vi "XIPIN_AXI_BFM_Cores_5_0.vi"   [LabVIEW 2017]
doc: "Cadence Axi BFM Cores\n------------------------------------\n<b>Need License</b> : Yes\n<b>Interface</b> : AXI4 AXI4-Stream"
uses:
  <vilib>/rvi/XilinxIP/XIPIN_XNode/niFpgaXIPIN.xnode
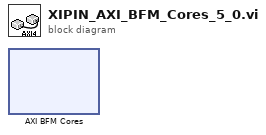
[diagram p0: block diagram]
diagram:
  n1 = xnode ("AXI BFM Cores")() -> ()
